vi "MHC-Serial Receive Test.vi"() -> ()   [LabVIEW 2020]
uses:
  <vilib>/Analysis/NI_AALBase.lvlib
  <vilib>/Analysis/baseanly.llb/Mean (DBL).vi
panel:
  out "Chart":cluster{"Speed":dbl, dbl}(graph)
  out "Speed 2":dbl format="%.2f mm/s"
  out "Speed":dbl format="%.2f mm/s"
  out "error out":errorcluster
  out "Phi":dbl format="%.0f °"
  out "R":dbl format="%.0f mm"
  out "time":string
  out "fps":dbl
  out "return count":u32
  in  "stop":bool
  out "Receive":string
  in  "VISA resource name":refnum<visa-resource-name>="COM7"
  in  "flow control":u16(ring)=2 items=["None"=0, "XON/XOFF"=1, "RTS/CTS"=2, "DTR/DSR"=4]
  in  "stop bits":u16(ring)=10 items=["1.0"=10, "1.5"=15, "2.0"=20]
  in  "parity":u16(ring) items=["None", "Odd", "Even", "Mark", "Space"]
  in  "data bits":u16=8 min=5 max=8 step=1
  in  "baud rate":u32=115200
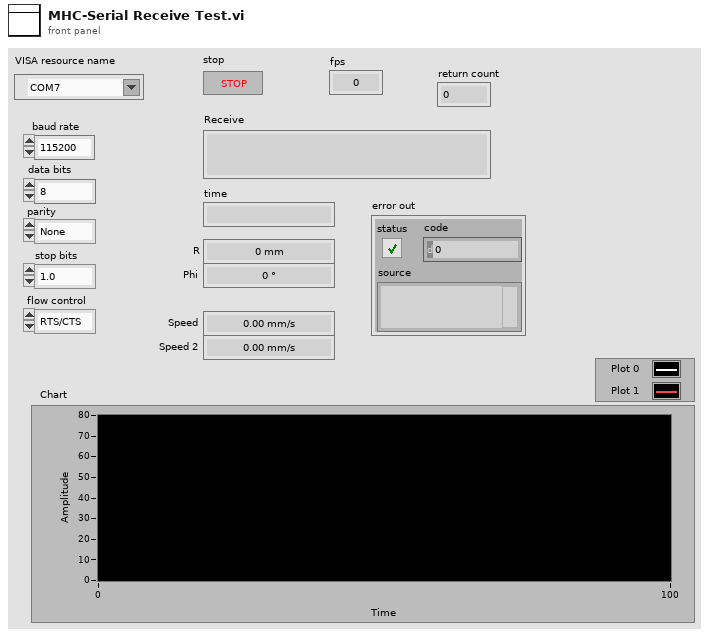
[diagram p1: front panel]
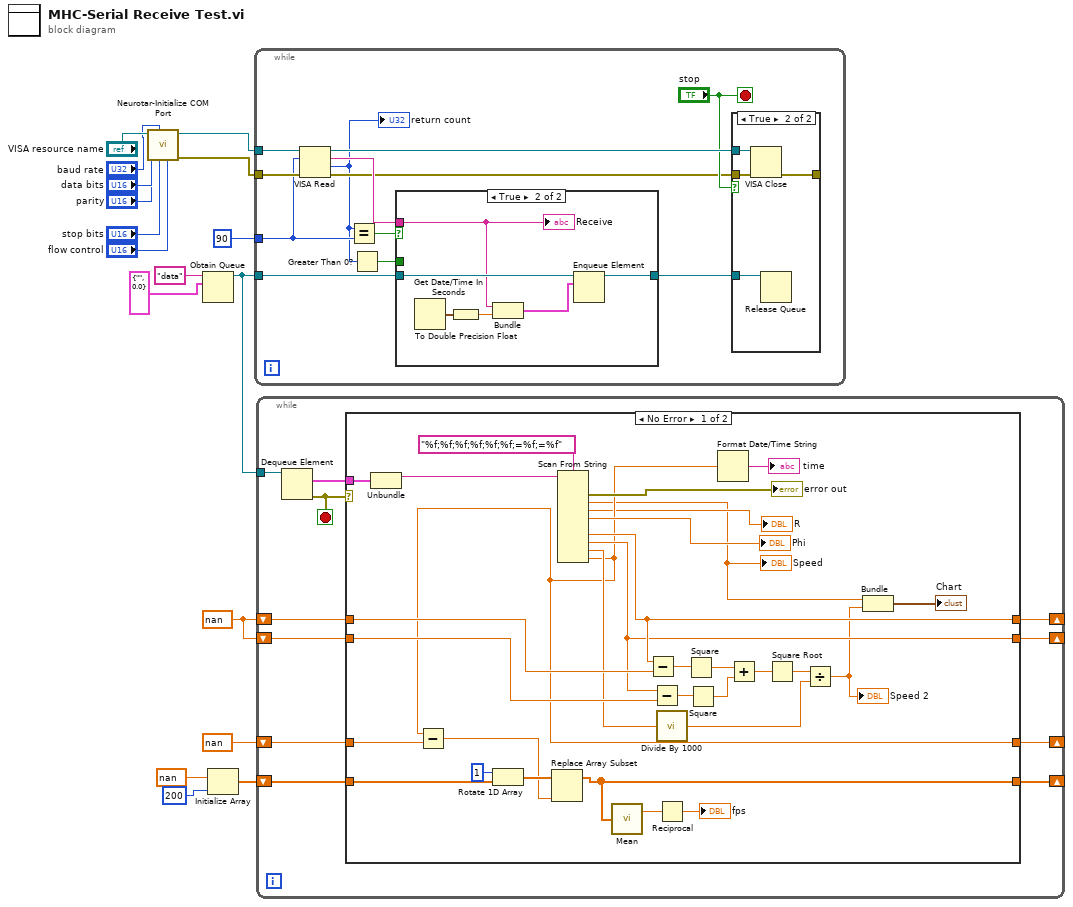
[diagram p0: block diagram]
diagram:
  w1 = nan
  n1 = call "Neurotar-Initialize COM Port.vi"("flow control"="flow control", "stop bits"="stop bits", "baud rate"="baud rate", "parity"="parity", "data bits"="data bits", "VISA Refnum in"="VISA resource name") -> ("error out"=w16:errorcluster, "VISA Refnum out"=w17:refnum<visa-resource-name>)  [unwired: 4 in]
  n2 = Obtain Queue(name (unnamed)="data", element data type=cluster{string, dbl} {"", 0.0}) -> (queue out=w7:refnum<queue>)  [unwired: 3 in, 2 out]
  n3 = Initialize Array(nan ("element"), 200 ("dimension size")) -> (w4:dbl[])
  n4 = while {
    tunnel: w17 -> [w27]
    tunnel: w16 -> [w26]
    tunnel: w7 -> [w23]
    tunnel: u32 90 ("byte count") -> [w20]
    stop <- "stop" stop-if-true
    n5 = VISA Read(VISA resource name=w27, byte count=w20, error in (no error)=w26) -> (VISA resource name out=w29:refnum<visa-resource-name>, read buffer=w28:string, return count=w19:u32, error out=w24:errorcluster)
    "return count" <- w19
    n6 = Equal?(x=w19, y=w20) -> (x = y?=w21:bool)
    n7 = Greater Than 0?(x=w19) -> (x > 0?=w18:bool)
    n8 = case shown="True" w21 {
      tunnel: w28 -> [_ w33]
      tunnel: w23 -> [w30 w36]
      tunnel: [w30 w32] -> w22
      tunnel: w18 -> [_ _]
      frame False {
      }
      frame True {
        n9 = Get Date/Time In Seconds() -> (seconds since 1Jan1904=w35:timestamp)
        n10 = To Double Precision Float(number=w35) -> (double precision float=w34:dbl)
        n11 = Bundle("read buffer"=w33, w34) -> (w31:cluster{"read buffer":string, dbl})  [unwired: 1 in]
        n12 = Enqueue Element(queue=w36, element=w31) -> (queue out=w32:refnum<queue>)  [unwired: 2 in, 2 out]
        "Receive" <- w33
      }
    }
    n13 = case shown="True" "stop" {
      tunnel: w29 -> [_ w40]
      tunnel: w24 -> [_ w39]
      tunnel: w22 -> [_ w38]
      tunnel: [_ w37] -> _
      frame False {
      }
      frame True {
        n14 = VISA Close(VISA resource name=w40, error in (no error)=w39) -> (error out=w37:errorcluster)
        n15 = Release Queue(queue=w38) -> ()  [unwired: 2 in, 3 out]
      }
    }
  }
  n16 = while {
    tunnel: w7 -> [w51]
    shift-right: [w47] -> _
    shift-left: w4 -> [w48]
    shift-right: [w45] -> _
    shift-left: nan -> [w46]
    shift-right: [w42] -> _
    shift-left: w1 -> [w44]
    shift-right: [w41] -> _
    shift-left: w1 -> [w43]
    stop <- w50 stop-if-true
    n17 = Dequeue Element(queue=w51) -> (element=w49:cluster{string, dbl}, error out=w50:errorcluster)  [unwired: 2 in, 2 out]
    n18 = case shown="No Error" w50 {
      tunnel: w49 -> [w82 _]
      tunnel: w48 -> [w80 w86]
      tunnel: [w76 w86] -> w47
      tunnel: w46 -> [w81 w85]
      tunnel: [w54 w85] -> w45
      tunnel: w44 -> [w67 w84]
      tunnel: w43 -> [w65 w83]
      tunnel: [w68 w84] -> w42
      tunnel: [w66 w83] -> w41
      frame No Error {
        n19 = Unbundle(w82) -> (w73:string)  [unwired: 1 out]
        n20 = Rotate 1D Array(1:w80, 2:1 ("n")) -> (0:w78:dbl[])
        n21 = Scan From String(format string="%f;%f;%f;%f;%f;%f;=%f;=%f", input string=w73) -> (error out=→"error out":errorcluster, output 1=w52:dbl, output 2=→"R":dbl, output 3=→"Phi":dbl, output 5=w68:dbl, output 6=w66:dbl, output 7=w58:dbl, output 8=w54:dbl)  [unwired: 11 in, 2 out]
        "Speed" <- w52
        n22 = Subtract(x=w54, y=w81) -> (x-y=w77:dbl)
        n23 = Replace Array Subset(array=w78, new element=w77) -> (w76:dbl[])  [unwired: 1 in]
        n24 = call-poly <vilib>:"Mean.vi"("X"=w76) -> ("mean"=w75:dbl)  [unwired: 1 out]
        n25 = Subtract(x=w68, y=w67) -> (x-y=w64:dbl)
        n26 = Subtract(x=w66, y=w65) -> (x-y=w59:dbl)
        n27 = call "Divide By 1000.vi"("X"=w58) -> ("X/1000"=w57:dbl)
        n28 = Reciprocal(x=w75) -> (1/x=→"fps":dbl)
        n29 = Square(x=w64) -> (x^2=w63:dbl)
        n30 = Square(x=w59) -> (x^2=w62:dbl)
        n31 = Format Date/Time String(seconds (now)=w54) -> (date/time string=→"time":string)  [unwired: 2 in]
        n32 = Add(x=w63, y=w62) -> (x+y=w61:dbl)
        n33 = Square Root(x=w61) -> (sqrt(x)=w60:dbl)
        n34 = Divide(x=w60, y=w57) -> (x/y=w56:dbl)
        "Speed 2" <- w56
        n35 = Bundle("Speed"=w52, w56) -> (→"Chart":cluster{"Speed":dbl, dbl})  [unwired: 1 in]
      }
      frame Error {
      }
    }
  }
